vi "Catapult Control Simulator.vi"() -> ()   [LabVIEW 2015]
uses:
  <userlib>/836 Library/Pneumatics/Catapult/836_CatapultActions.ctl
  <userlib>/836 Library/Pneumatics/Catapult/Catapult Configuration.ctl
  <vilib>/Rock Robotics/WPI/Solenoid/WPI_SolenoidChannel.ctl
  <vilib>/Rock Robotics/WPI/Solenoid/WPI_SolenoidOpenSingle.vi
panel:
  in  "Catapult Configuration":T1={"Time Forward"=3000, "Time Back"=2000, "Digital Forward Samples"=400, "Digital Backward Samples"=300, "Analog Forward Settling Time"=2000, "Analog Backward Settling Time"=3000, "Analog Forward Threshold"=4.0, "Analog Backward Threshold"=1.0}
  in  "Second Action":T2=enum."Retract Digital"
  in  "First Action":T2=enum."Fire Timed"
  out "Numeric":i32
  out "Action Complete":bool=TRUE
  out "Forward":bool
  in  "Sensor Analog Status":sgl(knob)=5.0 scale=0.0..5.0
  in  "Sensor Digital Status":bool
  in  "Step":bool
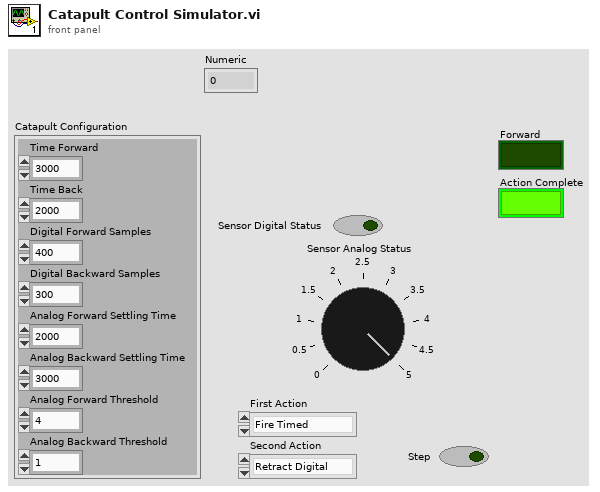
[diagram p1: front panel]
types:
  T1 = typedef "Catapult Configuration.ctl" = cluster{"Time Forward":u32, "Time Back":u32, "Digital Forward Samples":u32, "Digital Backward Samples":u32, "Analog Forward Settling Time":u32, "Analog Backward Settling Time":u32, "Analog Forward Threshold":sgl, "Analog Backward Threshold":sgl}
  T2 = typedef "836_CatapultActions.ctl" = enum8{"Fire", "Fire Timed", "Fire Analog", "Fire Digital", "Retract", "Retract Timed", "Retract Analog", "Retract Digital", "Hold", "Toggle", "Toggle Timed", "Toggle Analog", "Toggle Digital"}
  T3 = typedef "WPI_SolenoidChannel.ctl" = enum8{"Solenoid 0", "Solenoid 1", "Solenoid 2", "Solenoid 3", "Solenoid 4", "Solenoid 5", "Solenoid 6", "Solenoid 7", "Invalid"}
  T4 = typedef "WPI_SolenoidDevRef.ctl" = cluster{"DevStatus":errorcluster, "Pneumatics Control Module":u8, "Forward Solenoid Channel":T3, "Reverse Solenoid Channel":T3}
  T5 = typedef "836_CatapultDevRef.ctl" = cluster{"Catapult State Reference":refnum<data-value>, "SolenoidDevRef":T4, "Catapult Configuration Reference":refnum<data-value>}
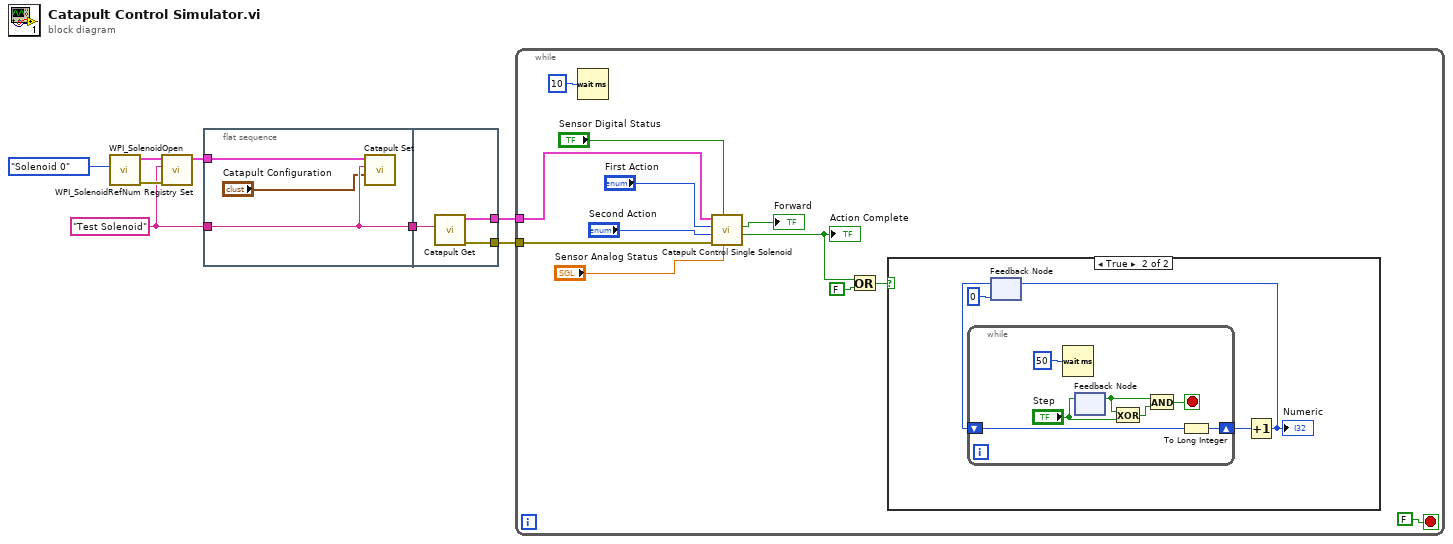
[diagram p0: block diagram]
diagram:
  w4 = "Test Solenoid" ("DevRef")
  n1 = call-poly <vilib>:"WPI_SolenoidOpen.vi"("Solenoid Channel"=WPI_SolenoidChannel."Solenoid 0") -> ("error out"=w6:errorcluster, "SolenoidDevRef"=w7:T4)  [unwired: 9 in]
  n2 = call <vilib>:"WPI_SolenoidRefNum Registry Set.vi"("error in (no error)"=w6, "refnum name"=w4, "SolenoidDevRef"=w7) -> ("SolenoidDevRef"=w5:T4)  [unwired: 7 in, 1 out]
  n3 = flat-sequence {
    tunnel: w4 -> [w11]
    tunnel: [w11] -> w8
    tunnel: w5 -> [w10]
    tunnel: [w14] -> w1
    tunnel: w8 -> [w13]
    tunnel: [w12] -> w2
    frame #0 {
      n4 = call <userlib>:"Catapult Set.vi"("Catapult Configuration"="Catapult Configuration", "DevRef"=w11, "SolenoidDevRef"=w10) -> ()  [unwired: 8 in, 1 out]
    }
    frame #1 {
      n5 = call <userlib>:"Catapult Get.vi"("DevRef"=w13) -> ("Error Out"=w14:errorcluster, "CatapultDevRefOut"=w12:T5)  [unwired: 9 in]
    }
  }
  n6 = while {
    tunnel: w2 -> [w21]
    tunnel: w1 -> [w18]
    stop <- FALSE stop-if-true
    n7 = Wait (ms)(milliseconds to wait=u32 10) -> ()  [unwired: 1 out]
    n8 = call <userlib>:"Catapult Control Single Solenoid.vi"("Sensor Analog Status"="Sensor Analog Status", "Sensor Digital Status"="Sensor Digital Status", "Error In"=w18, "Second Action"="Second Action", "First Action"="First Action", "CatapultDevRefIn"=w21) -> ("Action Complete"=w16:bool, "Solenoid Position"=→"Forward":bool)  [unwired: 3 in, 1 out]
    "Action Complete" <- w16
    n9 = Or(x=w16, y=FALSE) -> (x .or. y?=w17:bool)
    n10 = case shown="True" w17 {
      frame False {
      }
      frame True {
        n11 = feedback #1(0) -> (w29:i32)
        n12 = while {
          shift-right: [w33] -> w30
          shift-left: w29 -> [w32]
          stop <- w34 stop-if-true
          n13 = Wait (ms)(milliseconds to wait=u32 50) -> ()  [unwired: 1 out]
          n14 = feedback-in #2("Step") -> ()
          n15 = feedback #2() -> (w35:bool)  [unwired: 1 in]
          n16 = Exclusive Or(1:"Step", 2:w35) -> (0:w36:bool)
          n17 = And(x=w35, y=w36) -> (x .and. y?=w34:bool)
          n18 = To Long Integer(number=w32) -> (32bit integer=w33:i32)
        }
        n19 = Increment(x=w30) -> (x+1=w27:i32)
        "Numeric" <- w27
        n20 = feedback-in #1(w27) -> ()
      }
    }
  }
